vi "nmt_master_command.vi"(10 "node":u8, 11 "cs":u8) -> ()   [LabVIEW 2011]
uses:
  canopen_dll_master.dll
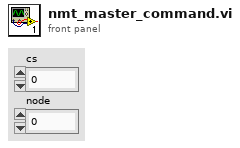
[diagram p1: front panel]
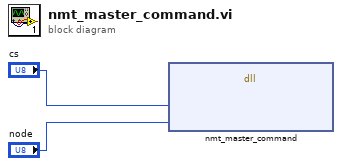
[diagram p0: block diagram]
diagram:
  n1 = dll-call lib="canopen_dll_master.dll" fn="nmt_master_command"("cs"="cs", "node"="node") -> ()  [unwired: 6 in, 2 out]
